vi "设置.vi"(6 "环境设定out":enum16{"不做控制", "清凉夏日", "温暖冬日", "自定义"}(ring), 9 "输出数值":cluster{"温度阈值":dbl, "亮度阈值":dbl, "电源阈值":dbl}, 10 "消息":T1, 11 "timed out?":bool) -> (3 "写入缓冲区":string)   [LabVIEW 2012]
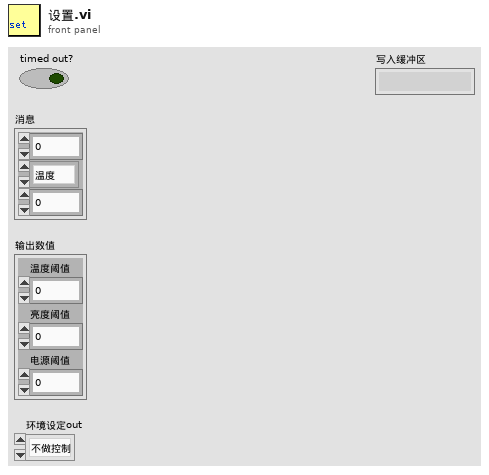
[diagram p1: front panel]
types:
  T1 = cluster{i32, enum16{"温度", "亮度", "电量", "连接质量"}, sgl}
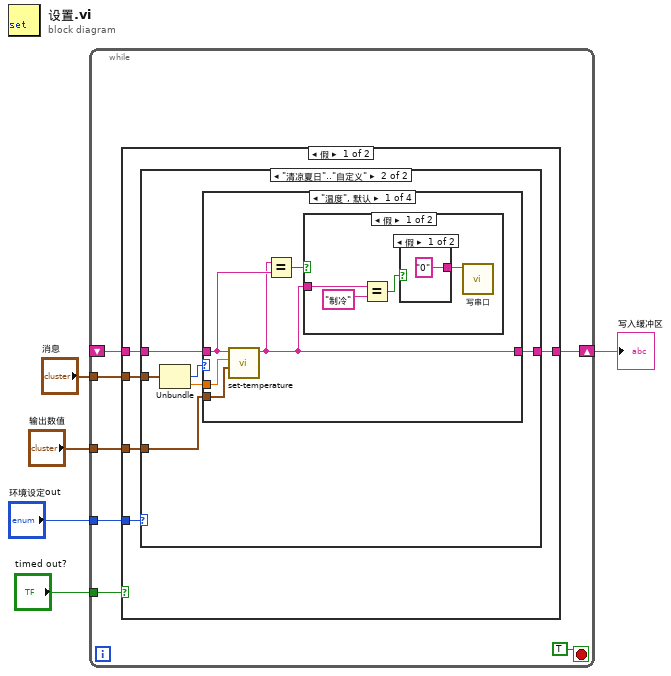
[diagram p0: block diagram]
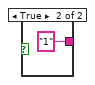
[diagram p3: hidden frame]
diagram:
  n1 = while {
    tunnel: "环境设定out" -> [w12]
    tunnel: "输出数值" -> [w11]
    tunnel: "消息" -> [w10]
    tunnel: "timed out?" -> [w9]
    shift-right: [w7] -> w1
    shift-left: _ -> [w6]
    stop <- TRUE stop-if-true
    n2 = case shown="假" w9 {
      tunnel: w10 -> [w15 _]
      tunnel: w11 -> [w16 _]
      tunnel: w12 -> [w17 _]
      tunnel: [w14 w39] -> w7
      tunnel: w6 -> [w13 w39]
      frame False {
        n3 = case shown="\"清凉夏日\"..\"自定义\"" w17 {
          tunnel: w16 -> [_ w22]
          tunnel: w15 -> [_ w24]
          tunnel: [w18 w20] -> w14
          tunnel: w13 -> [w18 w19]
          frame "不做控制", Default {
          }
          frame "清凉夏日".."自定义" {
            n4 = Unbundle(w24) -> (w23:enum16{"温度", "亮度", "电量", "连接质量"}, w21:sgl)  [unwired: 1 out]
            n5 = case shown="\"温度\", 默认" w23 {
              tunnel: w22 -> [w29 _ _ _]
              tunnel: w21 -> [w28 _ _ _]
              tunnel: [w25 w36 w37 w38] -> w20
              tunnel: w19 -> [w27 w36 w37 w38]
              frame "温度", Default {
                n6 = call "set-temperature.vi"("输出数值"=w29, "数值"=w28, "字符串输入"=w27) -> ("字符串输出"=w25:string)  [unwired: 8 in]
                n7 = Equal?(x=w25, y=w27) -> (x = y?=w26:bool)
                n8 = case shown="假" w26 {
                  tunnel: w25 -> [w33 _]
                  frame False {
                    n9 = Equal?(x=w33, y="制冷") -> (x = y?=w31:bool)
                    n10 = case shown="假" w31 {
                      tunnel: ["0" "1"] -> w30
                      frame False {
                      }
                      frame True {
                      }
                    }
                    n11 = call "写串口.vi"("写入缓冲区"=w30) -> ()  [unwired: 9 in, 2 out]
                  }
                  frame True {
                  }
                }
              }
              frame "亮度" {
              }
              frame "电量" {
              }
              frame "连接质量" {
              }
            }
          }
        }
      }
      frame True {
      }
    }
  }
  "写入缓冲区" <- w1
